vi "Set measurementservice_OCVData.vi"(7 "Complete Call (T)":bool=TRUE, 8 "error in (no error)":errorcluster, 10 "Message Data":T1, 11 "gRPCid":T4) -> (0 "error out":errorcluster)   [LabVIEW 2019, in "OCVTest.lvlib" / "OCVTest.lvclass"]
uses:
  OCVTest.lvclass
  gRPC lvSupport/Server API/typeDefs/grpcId.ctl
  measurementservice_OCVData_Data.ctl
  measurementservice_OCVRaw/measurementservice_OCVRaw_Data.ctl
  measurementservice_ErrorOut/measurementservice_ErrorOut_Data.ctl
  dcc74a39-081a-4bdd-860b-8ed792803c96.vi
  gRPC lvSupport/Server API/Server/Get Server DLL Path.vi
  <vilib>/Utility/error.llb/Error Cluster From Error Code.vi
  gRPC lvSupport/gprc-lvsupport.lvlib
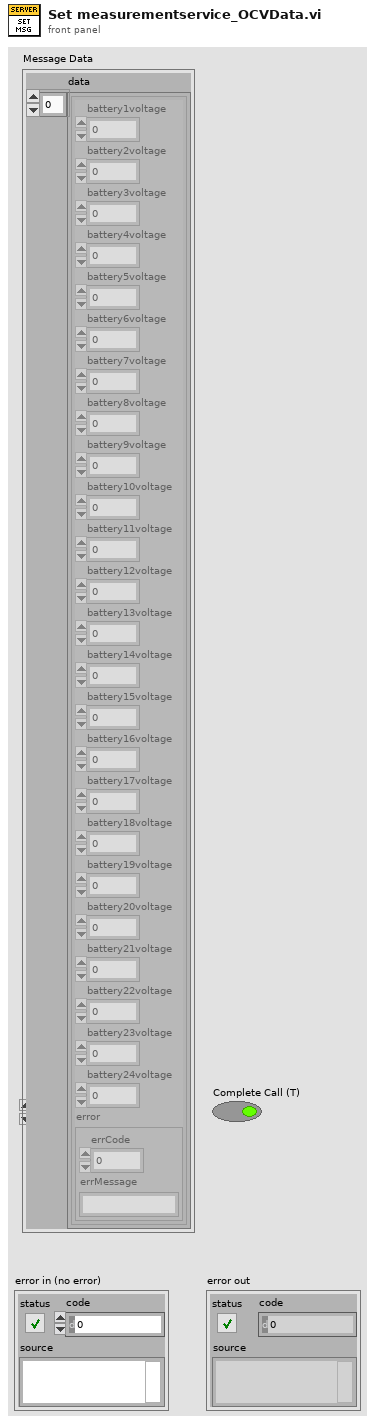
[diagram p1: front panel]
types:
  T1 = typedef "OCVTest.lvlib/OCVTest.lvclass/measurementservice_OCVData_Data.ctl" = cluster{"data":T2[]}
  T2 = typedef "OCVTest.lvlib/OCVTest.lvclass/measurementservice_OCVRaw_Data.ctl" = cluster{"battery1voltage":sgl, "battery2voltage":sgl, "battery3voltage":sgl, "battery4voltage":sgl, "battery5voltage":sgl, "battery6voltage":sgl, "battery7voltage":sgl, "battery8voltage":sgl, "battery9voltage":sgl, "battery10voltage":sgl, "battery11voltage":sgl, "battery12voltage":sgl, "battery13voltage":sgl, "battery14voltage":sgl, "battery15voltage":sgl, "battery16voltage":sgl, "battery17voltage":sgl, "battery18voltage":sgl, "battery19voltage":sgl, "battery20voltage":sgl, "battery21voltage":sgl, "battery22voltage":sgl, "battery23voltage":sgl, "battery24voltage":sgl, "error":T3}
  T3 = typedef "OCVTest.lvlib/OCVTest.lvclass/measurementservice_ErrorOut_Data.ctl" = cluster{"errCode":i32, "errMessage":string}
  T4 = typedef "OCVTest.lvlib/gprc-lvsupport.lvlib/grpcId.ctl" = u64
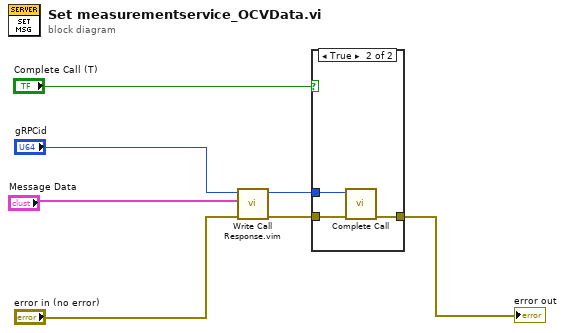
[diagram p0: block diagram]
diagram:
  n1 = call "Write Call Response.vim"("error in (no error)"="error in (no error)", "Response Data"="Message Data", "gRPCid in"="gRPCid") -> ("error out"=w4:errorcluster, "gRPCid"=w5:T4)  [unwired: 7 in]
  n2 = case shown="True" "Complete Call (T)" {
    tunnel: [w8 w11] -> w7
    tunnel: w5 -> [_ w10]
    tunnel: w4 -> [w8 w9]
    frame False {
    }
    frame True {
      n3 = call "Complete Call.vi"("gRPCid"=w10, "error in (no error)"=w9) -> ("error out"=w11:errorcluster)  [unwired: 8 in]
    }
  }
  "error out" <- w7
